vi "aft_Generate_Warning.vi"(6 "read coefficient? (F)":bool, 8 "error in (no error)":errorcluster, 9 "memory name":string, 10 "destination path":path, 11 "target ref":refnum<vi>) -> (0 "error out":errorcluster, 2 "continue":bool)   [LabVIEW 2017, in "NI_AdaptiveFilter.lvlib"]
uses:
  <vilib>/addons/Adaptive Filters/NI_AdaptiveFilter.lvlib
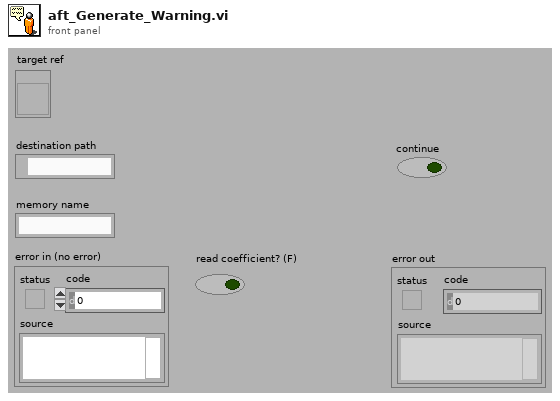
[diagram p1: front panel]
types:
  T1 = enum16{"Left Button", "Center Button", "Right Button", "Window Close"}
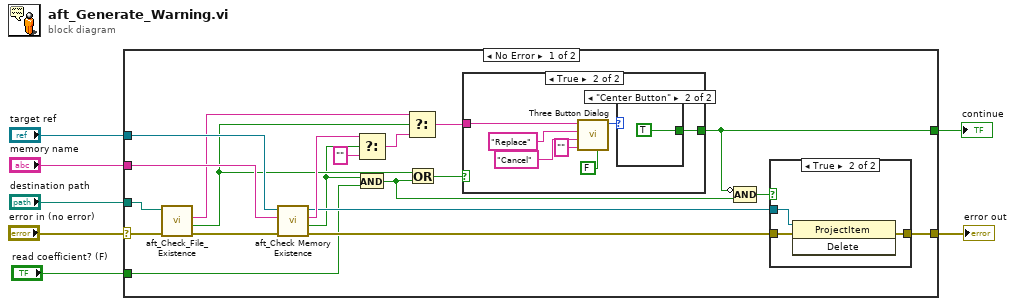
[diagram p0: block diagram]
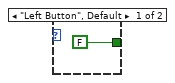
[diagram p4: hidden frame]
diagram:
  n1 = case shown="No Error" "error in (no error)" {
    selector: "error in (no error)" -> [w26 w41]
    tunnel: "destination path" -> [w27 _]
    tunnel: "target ref" -> [w22 _]
    tunnel: "memory name" -> [w21 _]
    tunnel: "read coefficient? (F)" -> [w9 _]
    tunnel: [w25 _] -> w2
    tunnel: [w23 w41] -> w1
    frame No Error {
      n2 = call <vilib>:"aft_Check_File_Existence.vi"("error in (no error)"=w26, "destination path"=w27) -> ("error out"=w20:errorcluster, "exists?"=w14:bool, "message"=w19:string)  [unwired: 3 in, 4 out]
      n3 = call <vilib>:"aft_Check Memory Existence.vi"("error in (no error)"=w20, "name"=w21, "target ref"=w22) -> ("error out"=w11:errorcluster, "exist?"=w10:bool, "msg"=w18:string, "memory ref"=w12:refnum<vi>)  [unwired: 5 in]
      n4 = Select(t=w18, s=w10, f="") -> (s? t:f=w16:string)
      n5 = And(x=w10, y=w9) -> (x .and. y?=w8:bool)
      n6 = Select(t=w19, s=w14, f=w16) -> (s? t:f=w15:string)
      n7 = Or(x=w14, y=w8) -> (x .or. y?=w13:bool)
      n8 = case shown="True" w13 {
        tunnel: w15 -> [_ w33]
        tunnel: [_ w32] -> w25
        frame False {
        }
        frame True {
          n9 = call <vilib>:"Three Button Dialog.vi"("Allow user to close window? (TRUE)"=FALSE, "Right Button Text (\"Cancel\")"="" ("Right Button Text (\"Cancel\")"), "Center Button Text (\"No\")"="Cancel" ("Center Button Text (\"No\")"), "Left Button Text (\"Yes\")"="Replace" ("Left Button Text (\"Yes\")"), "message"=w33) -> ("Which Button?"=w36:T1)  [unwired: 1 in, 5 out]
          n10 = case shown="\"Center Button\"" w36 {
            tunnel: [FALSE ("Allow user to close window? (TRUE)") TRUE ("Allow user to close window? (TRUE)")] -> w32
            frame "Left Button", Default {
            }
            frame "Center Button" {
            }
          }
        }
      }
      n11 = Compound Arithmetic op=AND(invert w25, w8) -> (w24:bool)
      n12 = case shown="True" w24 {
        tunnel: w11 -> [w28 w31]
        tunnel: w12 -> [_ w30]
        tunnel: [w28 w29] -> w23
        frame False {
        }
        frame True {
          n13 = invoke class="ProjectItem" method="Delete"(reference=w30, error in=w31) -> (error out=w29:errorcluster)  [unwired: 1 in, 2 out]
        }
      }
    }
    frame Error {
    }
  }
  "error out" <- w1
  "continue" <- w2
